vi "VI Tree.vi"   [LabVIEW 2020, in "Associated Research 78XX Series.lvlib"]
doc: "This instrument driver supports the Associated Power Technologies \"6000 Series Automated AC Power Source\".\n<B>Model Number</B> : 6005, 6010, 6020, 6040.\n\nThe VI Tree displays all the user-callable VIs of the instrument driver in an organized table.\n\nCreated By:\nAssociated Power Technologies, Inc. \n1142 S. Diamond Bar Blvd # 106 \nDiamond Bar , CA 91765 \n\nToll Free: 1-877-322-7693\nPhone: 1-909-860-1646\nFax: 1-909-860-2727\nEmail: info@aspowertechnologies.com"
uses:
  <instrlib>/Associated Research 78XX Series/Associated Research 78XX Series.lvlib
panel:
  # "Associated Research, Inc. \n13860 W. Laurel Drive \nLake Forest, IL 60045 \n\nToll Free:  1-800-858-8378\nPhone:      1-847-367-4077\nFax:          1-847-367-4080\nEmail:        info@arisafety.com"
  # "Please see diagram for ARI 78XX Driver VI Tree"
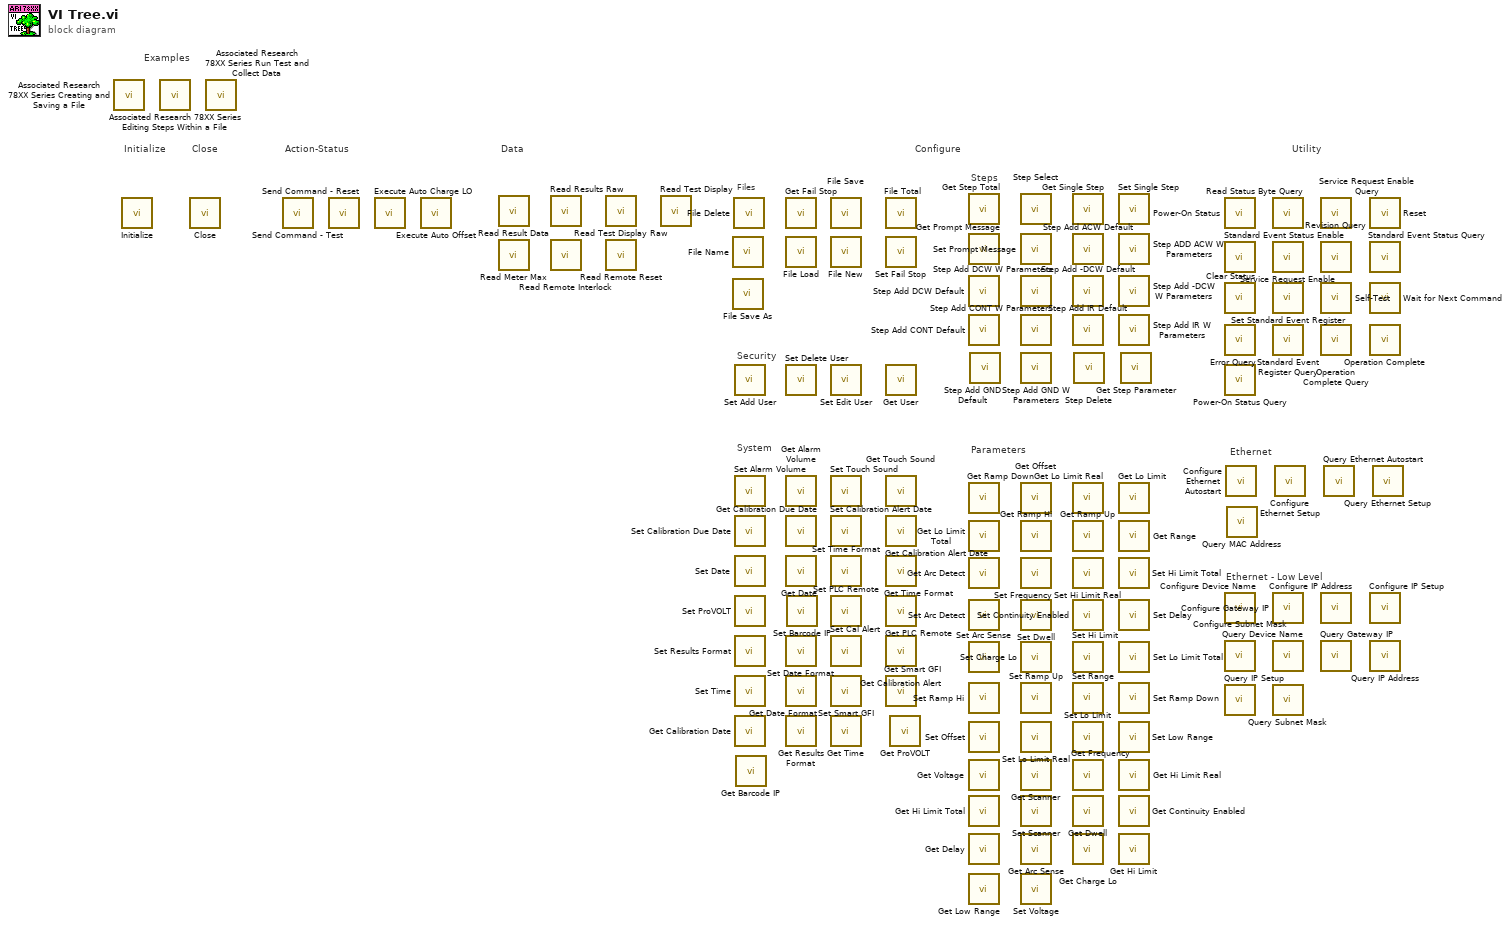
[diagram p0: block diagram]
diagram:
  # "Examples"
  # "Ethernet - Low Level"
  # "Ethernet"
  # "Data"
  # "System"
  # "Steps"
  # "Security"
  # "Parameters"
  # "Files"
  # "Configure"
  # "Utility"
  # "Action-Status"
  # "Close"
  # "Initialize"
  n1 = call <instrlib>:"Associated Research 78XX Series Creating and Saving a File.vi"() -> ()  [unwired: 11 in, 1 out]
  n2 = call <instrlib>:"Initialize.vi"() -> ()  [unwired: 13 in, 3 out]
  n3 = call <instrlib>:"Associated Research 78XX Series Editing Steps Within a File.vi"() -> ()  [unwired: 11 in, 1 out]
  n4 = call <instrlib>:"Close.vi"() -> ()  [unwired: 15 in, 1 out]
  n5 = call <instrlib>:"Associated Research 78XX Series Run Test and Collect Data.vi"() -> ()  [unwired: 11 in, 1 out]
  n6 = call <instrlib>:"Send Command - Test.vi"() -> ()  [unwired: 14 in, 2 out]
  n7 = call <instrlib>:"Send Command - Reset.vi"() -> ()  [unwired: 14 in, 2 out]
  n8 = call <instrlib>:"Execute Auto Charge LO.vi"() -> ()  [unwired: 14 in, 2 out]
  n9 = call <instrlib>:"Execute Auto Offset.vi"() -> ()  [unwired: 14 in, 2 out]
  n10 = call <instrlib>:"Read Result Data.vi"() -> ()  [unwired: 13 in, 3 out]
  n11 = call <instrlib>:"Read Meter Max.vi"() -> ()  [unwired: 8 in, 4 out]
  n12 = call <instrlib>:"Read Results Raw.vi"() -> ()  [unwired: 13 in, 3 out]
  n13 = call <instrlib>:"Read Remote Interlock.vi"() -> ()  [unwired: 13 in, 3 out]
  n14 = call <instrlib>:"Read Test Display Raw.vi"() -> ()  [unwired: 13 in, 3 out]
  n15 = call <instrlib>:"Read Remote Reset.vi"() -> ()  [unwired: 13 in, 3 out]
  n16 = call <instrlib>:"Read Test Display.vi"() -> ()  [unwired: 13 in, 3 out]
  n17 = call <instrlib>:"File Name.vi"() -> ()  [unwired: 13 in, 3 out]
  n18 = call <instrlib>:"File Save As.vi"() -> ()  [unwired: 14 in, 2 out]
  n19 = call <instrlib>:"File Delete.vi"() -> ()  [unwired: 14 in, 2 out]
  n20 = call <instrlib>:"Set Add User.vi"() -> ()  [unwired: 10 in, 2 out]
  n21 = call <instrlib>:"Set Alarm Volume.vi"() -> ()  [unwired: 10 in, 2 out]
  n22 = call <instrlib>:"Set Calibration Due Date.vi"() -> ()  [unwired: 10 in, 2 out]
  n23 = call <instrlib>:"Set Date.vi"() -> ()  [unwired: 10 in, 2 out]
  n24 = call <instrlib>:"Set ProVOLT.vi"() -> ()  [unwired: 10 in, 2 out]
  n25 = call <instrlib>:"Set Results Format.vi"() -> ()  [unwired: 14 in, 2 out]
  n26 = call <instrlib>:"Set Time.vi"() -> ()  [unwired: 10 in, 2 out]
  n27 = call <instrlib>:"Get Calibration Date.vi"() -> ()  [unwired: 9 in, 3 out]
  n28 = call <instrlib>:"Get Barcode IP.vi"() -> ()  [unwired: 13 in, 3 out]
  n29 = call <instrlib>:"Get Fail Stop.vi"() -> ()  [unwired: 9 in, 3 out]
  n30 = call <instrlib>:"File Load.vi"() -> ()  [unwired: 14 in, 2 out]
  n31 = call <instrlib>:"Set Delete User.vi"() -> ()  [unwired: 10 in, 2 out]
  n32 = call <instrlib>:"Get Alarm Volume.vi"() -> ()  [unwired: 9 in, 3 out]
  n33 = call <instrlib>:"Get Calibration Due Date.vi"() -> ()  [unwired: 9 in, 3 out]
  n34 = call <instrlib>:"Get Date.vi"() -> ()  [unwired: 9 in, 3 out]
  n35 = call <instrlib>:"Set Date Format.vi"() -> ()  [unwired: 10 in, 2 out]
  n36 = call <instrlib>:"Get Date Format.vi"() -> ()  [unwired: 9 in, 3 out]
  n37 = call <instrlib>:"Get Results Format.vi"() -> ()  [unwired: 9 in, 3 out]
  n38 = call <instrlib>:"Set Barcode IP.vi"() -> ()  [unwired: 14 in, 2 out]
  n39 = call <instrlib>:"File Save.vi"() -> ()  [unwired: 14 in, 2 out]
  n40 = call <instrlib>:"File New.vi"() -> ()  [unwired: 14 in, 2 out]
  n41 = call <instrlib>:"Set Edit User.vi"() -> ()  [unwired: 10 in, 2 out]
  n42 = call <instrlib>:"Set Touch Sound.vi"() -> ()  [unwired: 10 in, 2 out]
  n43 = call <instrlib>:"Set Calibration Alert Date.vi"() -> ()  [unwired: 10 in, 2 out]
  n44 = call <instrlib>:"Set Time Format.vi"() -> ()  [unwired: 10 in, 2 out]
  n45 = call <instrlib>:"Set PLC Remote.vi"() -> ()  [unwired: 10 in, 2 out]
  n46 = call <instrlib>:"Set Cal Alert.vi"() -> ()  [unwired: 10 in, 2 out]
  n47 = call <instrlib>:"Set Smart GFI.vi"() -> ()  [unwired: 10 in, 2 out]
  n48 = call <instrlib>:"Get Time.vi"() -> ()  [unwired: 9 in, 3 out]
  n49 = call <instrlib>:"File Total.vi"() -> ()  [unwired: 13 in, 3 out]
  n50 = call <instrlib>:"Set Fail Stop.vi"() -> ()  [unwired: 14 in, 2 out]
  n51 = call <instrlib>:"Get User.vi"() -> ()  [unwired: 6 in, 6 out]
  n52 = call <instrlib>:"Get Touch Sound.vi"() -> ()  [unwired: 9 in, 3 out]
  n53 = call <instrlib>:"Get Calibration Alert Date.vi"() -> ()  [unwired: 9 in, 3 out]
  n54 = call <instrlib>:"Get Time Format.vi"() -> ()  [unwired: 9 in, 3 out]
  n55 = call <instrlib>:"Get PLC Remote.vi"() -> ()  [unwired: 9 in, 3 out]
  n56 = call <instrlib>:"Get Calibration Alert.vi"() -> ()  [unwired: 9 in, 3 out]
  n57 = call <instrlib>:"Get Smart GFI.vi"() -> ()  [unwired: 8 in, 4 out]
  n58 = call <instrlib>:"Get ProVOLT.vi"() -> ()  [unwired: 9 in, 3 out]
  n59 = call <instrlib>:"Get Step Total.vi"() -> ()  [unwired: 13 in, 3 out]
  n60 = call <instrlib>:"Get Prompt Message.vi"() -> ()  [unwired: 13 in, 3 out]
  n61 = call <instrlib>:"Step Add DCW Default.vi"() -> ()  [unwired: 10 in, 2 out]
  n62 = call <instrlib>:"Step Add CONT Default.vi"() -> ()  [unwired: 10 in, 2 out]
  n63 = call <instrlib>:"Get Ramp Down.vi"() -> ()  [unwired: 9 in, 3 out]
  n64 = call <instrlib>:"Get Lo Limit Total.vi"() -> ()  [unwired: 9 in, 3 out]
  n65 = call <instrlib>:"Get Arc Detect.vi"() -> ()  [unwired: 9 in, 3 out]
  n66 = call <instrlib>:"Set Arc Detect.vi"() -> ()  [unwired: 10 in, 2 out]
  n67 = call <instrlib>:"Set Arc Sense.vi"() -> ()  [unwired: 10 in, 2 out]
  n68 = call <instrlib>:"Set Ramp Hi.vi"() -> ()  [unwired: 10 in, 2 out]
  n69 = call <instrlib>:"Set Offset.vi"() -> ()  [unwired: 10 in, 2 out]
  n70 = call <instrlib>:"Get Voltage.vi"() -> ()  [unwired: 9 in, 3 out]
  n71 = call <instrlib>:"Get Hi Limit Total.vi"() -> ()  [unwired: 9 in, 3 out]
  n72 = call <instrlib>:"Get Delay.vi"() -> ()  [unwired: 9 in, 3 out]
  n73 = call <instrlib>:"Get Low Range.vi"() -> ()  [unwired: 9 in, 3 out]
  n74 = call <instrlib>:"Step Add GND Default.vi"() -> ()  [unwired: 10 in, 2 out]
  n75 = call <instrlib>:"Step Select.vi"() -> ()  [unwired: 14 in, 2 out]
  n76 = call <instrlib>:"Set Prompt Message.vi"() -> ()  [unwired: 14 in, 2 out]
  n77 = call <instrlib>:"Step Add DCW W Parameters.vi"() -> ()  [unwired: 14 in, 2 out]
  n78 = call <instrlib>:"Step Add CONT W Parameters.vi"() -> ()  [unwired: 14 in, 2 out]
  n79 = call <instrlib>:"Step Add GND W Parameters.vi"() -> ()  [unwired: 14 in, 2 out]
  n80 = call <instrlib>:"Get Offset.vi"() -> ()  [unwired: 9 in, 3 out]
  n81 = call <instrlib>:"Get Ramp Hi.vi"() -> ()  [unwired: 9 in, 3 out]
  n82 = call <instrlib>:"Set Frequency.vi"() -> ()  [unwired: 10 in, 2 out]
  n83 = call <instrlib>:"Set Dwell.vi"() -> ()  [unwired: 10 in, 2 out]
  n84 = call <instrlib>:"Set Charge Lo.vi"() -> ()  [unwired: 10 in, 2 out]
  n85 = call <instrlib>:"Set Ramp Up.vi"() -> ()  [unwired: 10 in, 2 out]
  n86 = call <instrlib>:"Set Lo Limit Real.vi"() -> ()  [unwired: 10 in, 2 out]
  n87 = call <instrlib>:"Get Scanner.vi"() -> ()  [unwired: 9 in, 3 out]
  n88 = call <instrlib>:"Set Scanner.vi"() -> ()  [unwired: 10 in, 2 out]
  n89 = call <instrlib>:"Get Arc Sense.vi"() -> ()  [unwired: 9 in, 3 out]
  n90 = call <instrlib>:"Set Voltage.vi"() -> ()  [unwired: 10 in, 2 out]
  n91 = call <instrlib>:"Get Single Step.vi"() -> ()  [unwired: 9 in, 3 out]
  n92 = call <instrlib>:"Step Add ACW Default.vi"() -> ()  [unwired: 10 in, 2 out]
  n93 = call <instrlib>:"Step Add -DCW Default.vi"() -> ()  [unwired: 10 in, 2 out]
  n94 = call <instrlib>:"Step Add IR Default.vi"() -> ()  [unwired: 10 in, 2 out]
  n95 = call <instrlib>:"Get Lo Limit Real.vi"() -> ()  [unwired: 9 in, 3 out]
  n96 = call <instrlib>:"Get Ramp Up.vi"() -> ()  [unwired: 9 in, 3 out]
  n97 = call <instrlib>:"Set Hi Limit Real.vi"() -> ()  [unwired: 10 in, 2 out]
  n98 = call <instrlib>:"Set Continuity Enabled.vi"() -> ()  [unwired: 10 in, 2 out]
  n99 = call <instrlib>:"Set Hi Limit.vi"() -> ()  [unwired: 9 in, 2 out]
  n100 = call <instrlib>:"Set Range.vi"() -> ()  [unwired: 10 in, 2 out]
  n101 = call <instrlib>:"Set Lo Limit.vi"() -> ()  [unwired: 9 in, 2 out]
  n102 = call <instrlib>:"Get Frequency.vi"() -> ()  [unwired: 9 in, 3 out]
  n103 = call <instrlib>:"Get Dwell.vi"() -> ()  [unwired: 9 in, 3 out]
  n104 = call <instrlib>:"Get Charge Lo.vi"() -> ()  [unwired: 9 in, 3 out]
  n105 = call <instrlib>:"Step Delete.vi"() -> ()  [unwired: 14 in, 2 out]
  n106 = call <instrlib>:"Set Single Step.vi"() -> ()  [unwired: 14 in, 2 out]
  n107 = call <instrlib>:"Step ADD ACW W Parameters.vi"() -> ()  [unwired: 14 in, 2 out]
  n108 = call <instrlib>:"Step Add -DCW W Parameters.vi"() -> ()  [unwired: 14 in, 2 out]
  n109 = call <instrlib>:"Step Add IR W Parameters.vi"() -> ()  [unwired: 14 in, 2 out]
  n110 = call <instrlib>:"Get Lo Limit.vi"() -> ()  [unwired: 9 in, 3 out]
  n111 = call <instrlib>:"Get Range.vi"() -> ()  [unwired: 9 in, 3 out]
  n112 = call <instrlib>:"Set Hi Limit Total.vi"() -> ()  [unwired: 10 in, 2 out]
  n113 = call <instrlib>:"Set Delay.vi"() -> ()  [unwired: 14 in, 2 out]
  n114 = call <instrlib>:"Set Lo Limit Total.vi"() -> ()  [unwired: 10 in, 2 out]
  n115 = call <instrlib>:"Set Ramp Down.vi"() -> ()  [unwired: 10 in, 2 out]
  n116 = call <instrlib>:"Set Low Range.vi"() -> ()  [unwired: 10 in, 2 out]
  n117 = call <instrlib>:"Get Hi Limit Real.vi"() -> ()  [unwired: 9 in, 3 out]
  n118 = call <instrlib>:"Get Continuity Enabled.vi"() -> ()  [unwired: 9 in, 3 out]
  n119 = call <instrlib>:"Get Hi Limit.vi"() -> ()  [unwired: 9 in, 3 out]
  n120 = call <instrlib>:"Get Step Parameter.vi"() -> ()  [unwired: 13 in, 3 out]
  n121 = call <instrlib>:"Power-On Status.vi"() -> ()  [unwired: 14 in, 2 out]
  n122 = call <instrlib>:"Standard Event Status Enable.vi"() -> ()  [unwired: 14 in, 2 out]
  n123 = call <instrlib>:"Clear Status.vi"() -> ()  [unwired: 14 in, 2 out]
  n124 = call <instrlib>:"Error Query.vi"() -> ()  [unwired: 12 in, 4 out]
  n125 = call <instrlib>:"Power-On Status Query.vi"() -> ()  [unwired: 13 in, 3 out]
  n126 = call <instrlib>:"Configure Device Name.vi"() -> ()  [unwired: 14 in, 2 out]
  n127 = call <instrlib>:"Configure Subnet Mask.vi"() -> ()  [unwired: 14 in, 2 out]
  n128 = call <instrlib>:"Query IP Setup.vi"() -> ()  [unwired: 13 in, 3 out]
  n129 = call <instrlib>:"Configure Ethernet Autostart.vi"() -> ()  [unwired: 14 in, 2 out]
  n130 = call <instrlib>:"Query MAC Address.vi"() -> ()  [unwired: 13 in, 3 out]
  n131 = call <instrlib>:"Read Status Byte Query.vi"() -> ()  [unwired: 13 in, 3 out]
  n132 = call <instrlib>:"Service Request Enable.vi"() -> ()  [unwired: 14 in, 2 out]
  n133 = call <instrlib>:"Set Standard Event Register.vi"() -> ()  [unwired: 14 in, 2 out]
  n134 = call <instrlib>:"Standard Event Register Query.vi"() -> ()  [unwired: 13 in, 3 out]
  n135 = call <instrlib>:"Configure Gateway IP.vi"() -> ()  [unwired: 14 in, 2 out]
  n136 = call <instrlib>:"Query Device Name.vi"() -> ()  [unwired: 13 in, 3 out]
  n137 = call <instrlib>:"Query Subnet Mask.vi"() -> ()  [unwired: 13 in, 3 out]
  n138 = call <instrlib>:"Configure Ethernet Setup.vi"() -> ()  [unwired: 10 in, 2 out]
  n139 = call <instrlib>:"Service Request Enable Query.vi"() -> ()  [unwired: 13 in, 3 out]
  n140 = call <instrlib>:"Revision Query.vi"() -> ()  [unwired: 11 in, 5 out]
  n141 = call <instrlib>:"Self-Test.vi"() -> ()  [unwired: 12 in, 4 out]
  n142 = call <instrlib>:"Operation Complete Query.vi"() -> ()  [unwired: 13 in, 3 out]
  n143 = call <instrlib>:"Configure IP Address.vi"() -> ()  [unwired: 14 in, 2 out]
  n144 = call <instrlib>:"Query Gateway IP.vi"() -> ()  [unwired: 13 in, 3 out]
  n145 = call <instrlib>:"Query Ethernet Autostart.vi"() -> ()  [unwired: 13 in, 3 out]
  n146 = call <instrlib>:"Reset.vi"() -> ()  [unwired: 14 in, 2 out]
  n147 = call <instrlib>:"Standard Event Status Query.vi"() -> ()  [unwired: 13 in, 3 out]
  n148 = call <instrlib>:"Wait for Next Command.vi"() -> ()  [unwired: 14 in, 2 out]
  n149 = call <instrlib>:"Operation Complete.vi"() -> ()  [unwired: 14 in, 2 out]
  n150 = call <instrlib>:"Configure IP Setup.vi"() -> ()  [unwired: 14 in, 2 out]
  n151 = call <instrlib>:"Query IP Address.vi"() -> ()  [unwired: 13 in, 3 out]
  n152 = call <instrlib>:"Query Ethernet Setup.vi"() -> ()  [unwired: 5 in, 7 out]
